vi "wyciaga_nazwy_kanalow_z_grupy.vi"(7 "Group":string, 8 "error in (no error)":errorcluster, 11 "group/channel names":string[][](array[string])) -> (0 "error out":errorcluster, 1 "channel names":string[](array[string]))   [LabVIEW 2014]
doc: "Wyciąga nazwy kanałów z grupy o zadanej nazwie"
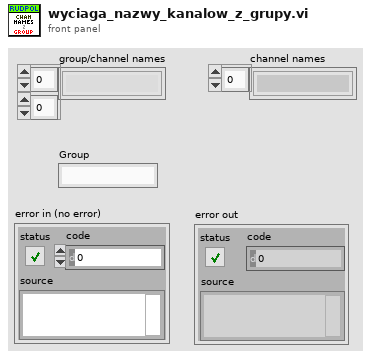
[diagram p1: front panel]
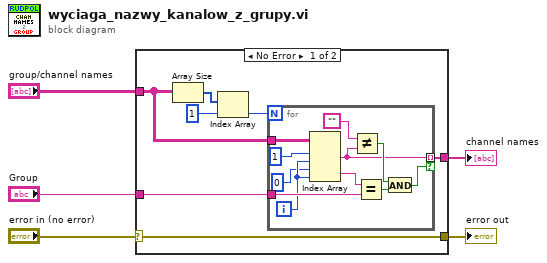
[diagram p0: block diagram]
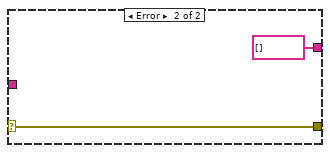
[diagram p2: hidden frame]
diagram:
  n1 = case shown="No Error" "error in (no error)" {
    selector: "error in (no error)" -> [w6 w24]
    tunnel: [w12 string[] []] -> w5
    tunnel: "Group" -> [w11 _]
    tunnel: "group/channel names" -> [w10 _]
    tunnel: [w6 w24] -> w1
    frame No Error {
      n2 = Array Size(array=w10) -> (size(s)=w8:i32[])
      n3 = Index Array(array=w8, index=1) -> (element=w7:i32)
      n4 = for {
        N: w7 -> [_]
        tunnel: w10 -> [w23]
        tunnel: w11 -> [w21]
        tunnel: [w17] -> w12 mode=indexing if=w16
        i -> [w15]
        n5 = Index Array(array=w23, index (row) #1=1 ("index"), index (col) #1=w15, index (row) #2=0 ("index"), index (col) #2=w15) -> (element #1=w17:string, element #2=w22:string)
        n6 = Not Equal?(x="", y=w17) -> (x != y?=w18:bool)
        n7 = Equal?(x=w22, y=w21) -> (x = y?=w20:bool)
        n8 = And(x=w18, y=w20) -> (x .and. y?=w16:bool)
      }
    }
    frame Error {
    }
  }
  "channel names" <- w5
  "error out" <- w1
